vi "Sinusoidal_Harmonic_Calculator_Sagar.vi"(8 "Phase":dbl, 9 "Amplitude (1/x)":dbl, 10 "Harmonic":dbl, 11 "Numeric in":dbl) -> (3 "Numeric out":dbl)   [LabVIEW 2022 SP3]
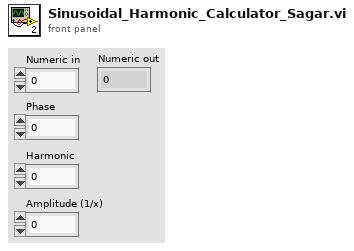
[diagram p1: front panel]
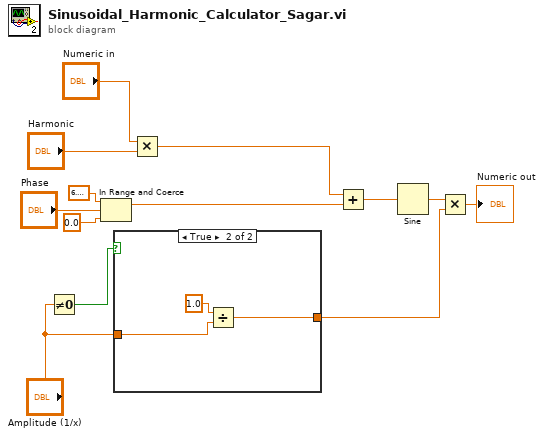
[diagram p0: block diagram]
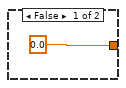
[diagram p2: hidden frame]
diagram:
  n1 = Not Equal To 0?(x="Amplitude (1/x)") -> (x != 0?=w3:bool)
  n2 = In Range and Coerce(upper limit=6.283185307179586, x="Phase", lower limit=0.0) -> (coerced(x)=w4:dbl)  [unwired: 1 out]
  n3 = case shown="True" w3 {
    tunnel: "Amplitude (1/x)" -> [_ w16]
    tunnel: [0.0 w15] -> w1
    frame False {
    }
    frame True {
      n4 = Divide(x=1.0, y=w16) -> (x/y=w15:dbl)
    }
  }
  n5 = Multiply(x="Numeric in", y="Harmonic") -> (x*y=w6:dbl)
  n6 = Add(x=w6, y=w4) -> (x+y=w5:dbl)
  n7 = Sine(x=w5) -> (sin(x)=w11:dbl)
  n8 = Multiply(x=w11, y=w1) -> (x*y=→"Numeric out":dbl)
